vi "CONTROLLER.vi"() -> ()   [LabVIEW 2013]
uses:
  base/CONTROLLER.lvclass
  View/base/VIEW.lvclass
  Model/base/MODEL.lvclass
panel:
  in  "Stop":bool
  out "error out":errorcluster
  in  "error in":errorcluster
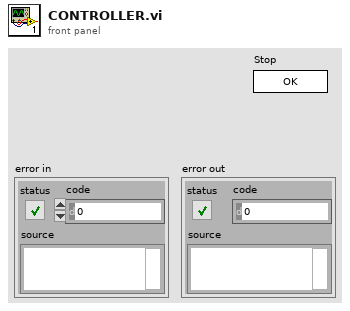
[diagram p1: front panel]
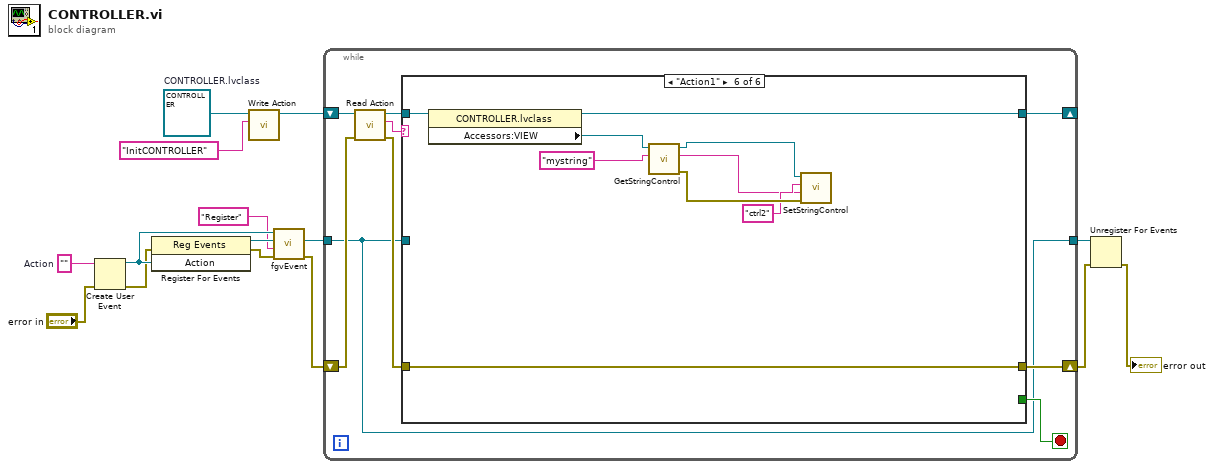
[diagram p0: block diagram]
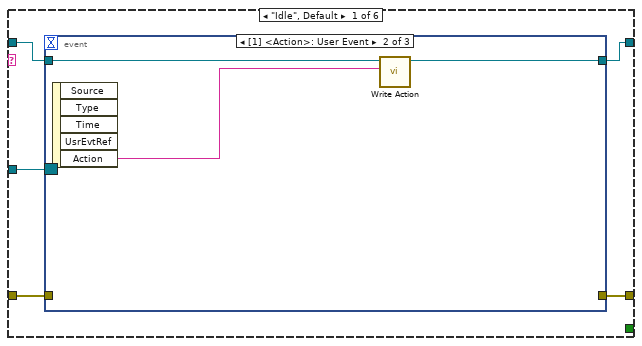
[diagram p2: hidden frame]
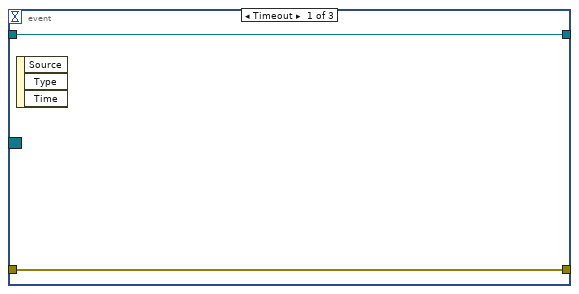
[diagram p3: hidden frame]
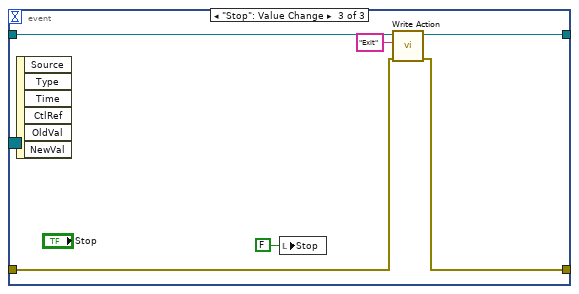
[diagram p4: hidden frame]
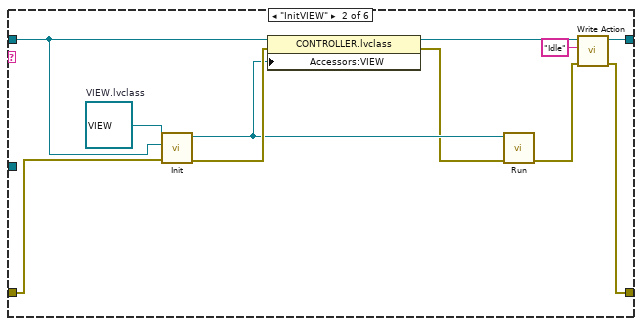
[diagram p5: hidden frame]
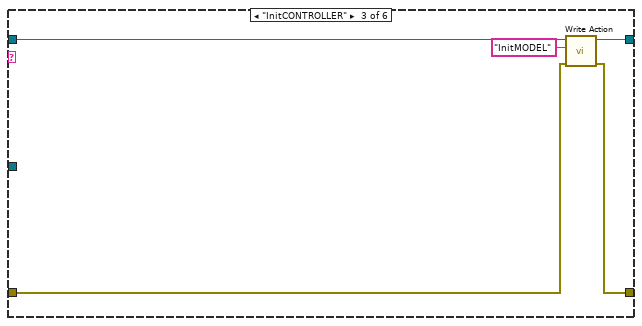
[diagram p6: hidden frame]
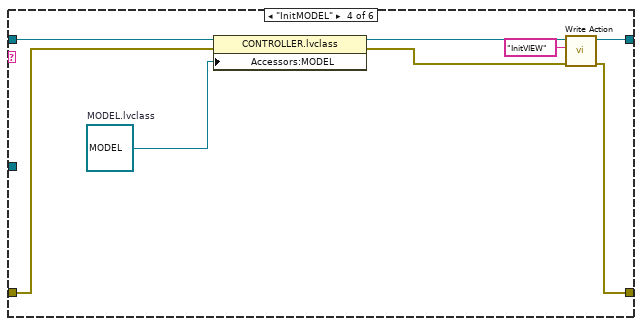
[diagram p7: hidden frame]
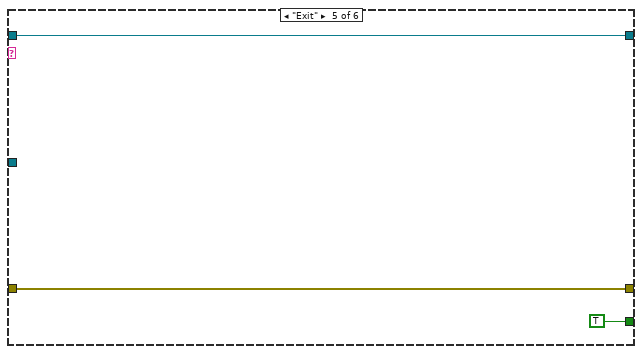
[diagram p8: hidden frame]
diagram:
  w12 = ""  # Action
  w15 = refnum<class "CONTROLLER.lvclass"> refnum  # CONTROLLER.lvclass
  n1 = Create User Event(user event datatype=w12, error in="error in") -> (user event=w7:refnum<user-event>, error out=w1:errorcluster)
  n2 = register-events(error in=w1, w7) -> (reference out=w8:refnum<event-registration>, error out=w4:errorcluster)  [unwired: 1 in]
  n3 = call-dynamic "Write Action.vi"("Action"="InitCONTROLLER", "CONTROLLER in"=w15) -> ("CONTROLLER out"=w14:refnum<class "CONTROLLER.lvclass">)  [unwired: 8 in, 1 out]
  n4 = call "fgvEvent.vi"("error in (no error)"=w4, "Cmd"="Register", "EventRefNum"=w8, "eventData"=w7) -> ("error out"=w3:errorcluster, "EventRefNum Out"=w5:refnum<event-registration>)  [unwired: 5 in, 1 out]
  n5 = while {
    shift-right: [w24] -> _
    shift-left: w14 -> [w23]
    shift-right: [w19] -> w11
    shift-left: w3 -> [w18]
    tunnel: w5 -> [w16]
    tunnel: [w16] -> w9
    stop <- w20 stop-if-true
    n6 = call-dynamic "Read Action.vi"("error in (no error)"=w18, "CONTROLLER in"=w23) -> ("error out"=w17:errorcluster, "Action"=w21:string, "CONTROLLER out"=w22:refnum<class "CONTROLLER.lvclass">)  [unwired: 7 in]
    n7 = case shown="\"Action1\"" w21 {
      tunnel: w22 -> [w25 w45 w56 w64 w67 w76]
      tunnel: [w26 w44 w55 w63 w67 w74] -> w24
      tunnel: [_ _ _ _ TRUE _] -> w20
      tunnel: [w28 w41 w53 w57 w65 w75] -> w19
      tunnel: w17 -> [w27 w49 w52 w59 w65 w75]
      tunnel: w16 -> [w29 _ _ _ _ _]
      frame "Idle", Default {
        n8 = event shown="[1] <Action>: User Event" {
          selector: w29 -> [_ _ _]
          dyn-events: _ -> [_ _ _]
          timeout: _ -> [_ _ _]
          tunnel: [w31 _ w36] -> w28
          tunnel: w27 -> [w31 _ w37]
          tunnel: [w30 w33 w39] -> w26
          tunnel: w25 -> [w30 w34 w40]
          event Timeout {
            n9 = event-data() -> ()  [unwired: 1 in, 3 out]
          }
          event User Event {
            n10 = event-data() -> ("Action"=w32:string)  [unwired: 1 in, 4 out]
            n11 = call-dynamic "Write Action.vi"("Action"=w32, "CONTROLLER in"=w34) -> ("CONTROLLER out"=w33:refnum<class "CONTROLLER.lvclass">)  [unwired: 8 in, 1 out]
          }
          event "Stop": Value Change {
            n12 = event-data() -> ()  [unwired: 1 in, 6 out]
            n13 = local write "Stop"(FALSE ("Stop")) -> ()
            n14 = call-dynamic "Write Action.vi"("error in (no error)"=w37, "Action"="Exit", "CONTROLLER in"=w40) -> ("error out"=w36:errorcluster, "CONTROLLER out"=w39:refnum<class "CONTROLLER.lvclass">)  [unwired: 7 in]
          }
        }
      }
      frame "InitVIEW" {
        w50 = refnum<class "VIEW.lvclass"> refnum  # VIEW.lvclass
        n15 = call-dynamic "Init.vi"("error in (no error)"=w49, "CONTROLLER"=w45, "VIEW in"=w50) -> ("error out"=w48:errorcluster, "VIEW out"=w47:refnum<class "VIEW.lvclass">)  [unwired: 7 in]
        n16 = property class="CONTROLLER.lvclass"(reference=w45, error in=w48, "Accessors:VIEW"=w47) -> (reference out=w51:refnum<class "CONTROLLER.lvclass">, error out=w46:errorcluster)
        n17 = call-dynamic "Run.vi"("error in (no error)"=w46, "VIEW in"=w47) -> ("error out"=w42:errorcluster)  [unwired: 8 in, 1 out]
        n18 = call-dynamic "Write Action.vi"("error in (no error)"=w42, "Action"="Idle", "CONTROLLER in"=w51) -> ("error out"=w41:errorcluster, "CONTROLLER out"=w44:refnum<class "CONTROLLER.lvclass">)  [unwired: 7 in]
      }
      frame "InitCONTROLLER" {
        n19 = call-dynamic "Write Action.vi"("error in (no error)"=w52, "Action"="InitMODEL", "CONTROLLER in"=w56) -> ("error out"=w53:errorcluster, "CONTROLLER out"=w55:refnum<class "CONTROLLER.lvclass">)  [unwired: 7 in]
      }
      frame "InitMODEL" {
        w60 = refnum<class "MODEL.lvclass"> refnum  # MODEL.lvclass
        n20 = property class="CONTROLLER.lvclass"(reference=w64, error in=w59, "Accessors:MODEL"=w60) -> (reference out=w61:refnum<class "CONTROLLER.lvclass">, error out=w58:errorcluster)
        n21 = call-dynamic "Write Action.vi"("error in (no error)"=w58, "Action"="InitVIEW", "CONTROLLER in"=w61) -> ("error out"=w57:errorcluster, "CONTROLLER out"=w63:refnum<class "CONTROLLER.lvclass">)  [unwired: 7 in]
      }
      frame "Exit" {
      }
      frame "Action1" {
        n22 = property class="CONTROLLER.lvclass"(reference=w76) -> (reference out=w74:refnum<class "CONTROLLER.lvclass">, "Accessors:VIEW"=w73:refnum<class "VIEW.lvclass">)  [unwired: 1 in, 1 out]
        n23 = call "GetStringControl.vi"("Name"="mystring", "VIEW in"=w73) -> ("error out"=w72:errorcluster, "Text.Text"=w68:string, "VIEW out"=w70:refnum<class "VIEW.lvclass">)  [unwired: 7 in]
        n24 = call "SetStringControl.vi"("error in (no error)"=w72, "Text.Text"=w68, "Name"="ctrl2", "VIEW in"=w70) -> ()  [unwired: 6 in, 2 out]
      }
    }
  }
  n25 = Unregister For Events(event registration refnum=w9, error in=w11) -> (error out=→"error out":errorcluster)
